vi "PCO_GetBufferStatus.vi"(8 "error in (no error)":errorcluster, 10 "sBufNr":i16, 11 "Handle":u64) -> (0 "error out":errorcluster, 1 "dwStatusDrv 0=noError":i32 format="%x", 2 "StatusDll":T1, 3 "Handle Out":u64, 4 "swStatusDll-raw":u32 format="%x", 5 "return type":u32 format="%x")   [LabVIEW 2011]
uses:
  SC2_Cam64.dll
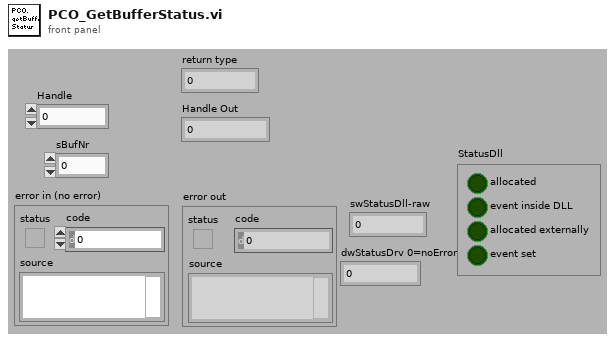
[diagram p1: front panel]
types:
  T1 = cluster{"allocated":bool, "event inside DLL":bool, "allocated externally":bool, "event set":bool}
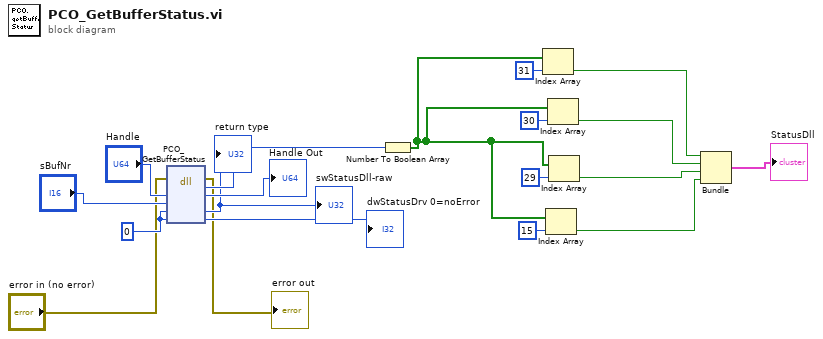
[diagram p0: block diagram]
diagram:
  w15 = 0
  n1 = dll-call lib="SC2_Cam*.*" fn="PCO_GetBufferStatus"(error in="error in (no error)", "Handle"="Handle", "sBufNr"="sBufNr", "swStatusDll"=w15, "dwStatusDrv"=w15) -> (error out=→"error out":errorcluster, "return type"=→"return type":u32, "Handle"=→"Handle Out":u64, "swStatusDll"=w13:u32, "dwStatusDrv"=→"dwStatusDrv 0=noError":i32)  [unwired: 3 in, 1 out]
  "swStatusDll-raw" <- w13
  n2 = Number To Boolean Array(number=w13) -> (Boolean array=w8:bool[])
  n3 = Index Array(array=w8, index=31) -> (element=w7:bool)
  n4 = Index Array(array=w8, index=15) -> (element=w4:bool)
  n5 = Index Array(array=w8, index=30) -> (element=w6:bool)
  n6 = Index Array(array=w8, index=29) -> (element=w5:bool)
  n7 = Bundle(w7, w6, w5, w4) -> (→"StatusDll":cluster{bool, bool, bool, bool})  [unwired: 1 out]
